vi "State Queue POP.vi"(7 "Default state":string="User action?", 8 "error in (no error)":errorcluster, 11 "State que in":T1[](array[typedef])) -> (0 "error out":errorcluster, 1 "Parameters":variant, 3 "State que out":T1[](array[typedef]), 4 "Not Exit?":bool, 5 "State case out":string)   [LabVIEW 2013, in "State Machine Lib.lvlib"]
doc: "Pops the next state off the state queue. Determines if the state is the exit state. Will catch errors and not pop the next state but returns the error state for error handeling.s"
uses:
  State Machine Lib.lvlib
  STATE cluster.ctl
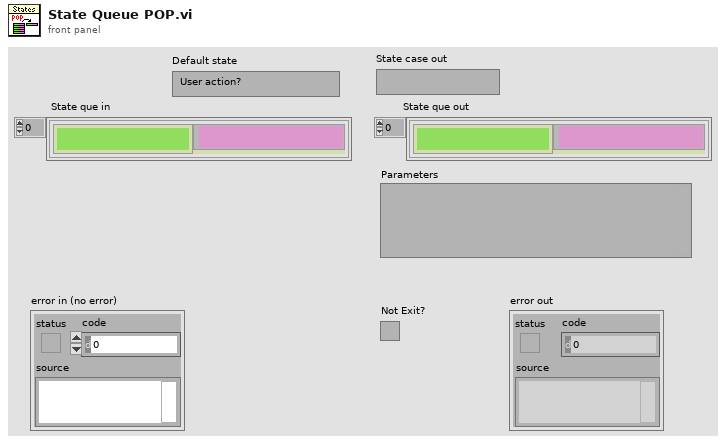
[diagram p1: front panel]
types:
  T1 = typedef "State Machine Lib.lvlib/STATE cluster.ctl" = cluster{"State":string, "Parameters":variant}
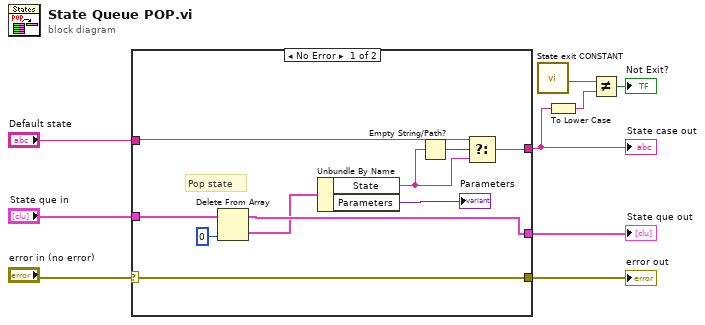
[diagram p0: block diagram]
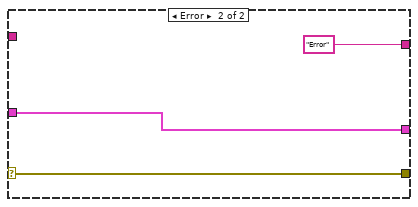
[diagram p2: hidden frame]
diagram:
  n1 = case shown="No Error" "error in (no error)" {
    selector: "error in (no error)" -> [w16 w20]
    tunnel: [w16 w20] -> w3
    tunnel: [w17 "Error"] -> w6
    tunnel: [w11 w22] -> w8
    tunnel: "State que in" -> [w12 w22]
    tunnel: "Default state" -> [w19 _]
    frame No Error {
      # "Pop state"
      n2 = Delete From Array(array=w12, index=0) -> (deleted portion=w10:T1, array with subset deleted=w11:T1[])  [unwired: 1 in]
      n3 = Unbundle By Name(w10) -> ("State"=w15:string, "Parameters"=→"Parameters":variant)
      n4 = Empty String/Path?(string/path=w15) -> (empty?=w18:bool)
      n5 = Select(t=w19, s=w18, f=w15) -> (s? t:f=w17:string)
    }
    frame Error {
    }
  }
  "State case out" <- w6
  "State que out" <- w8
  "error out" <- w3
  n6 = call "State exit CONSTANT.vi"() -> ("Exit state"=w1:string)
  n7 = To Lower Case(string=w6) -> (all lower case string=w5:string)
  n8 = Not Equal?(x=w1, y=w5) -> (x != y?=→"Not Exit?":bool)
